vi "CSV_Image_Data_Append.vi"(0 "input cluster":T2={"Pinch-valve"="Test Sample", "XLP 6000 Pump"="MRJ", "Camera1"="", "Camera2"="", "Img_Capt"=FALSE, "Actuator"=FALSE, "Pump"=FALSE, "Cam 1"=FALSE, "Cam 2"=FALSE, "Empty_Refill"=FALSE, "Crop"=FALSE, "Light intensity"=0, "Exposure Time"=0.0, "Sample Name"="", "Operator"="", "Calibration 1"=path "C:/Users/au540322/Desktop/IHS_Project/images/Debris/Debris_0/Debris_0_2019_06_01-23-32-49-686.PNG", "Calibration 2"=path "C:/Users/au540322/Desktop/IHS_Project/images/Debris/Debris_0/Debris_0_2019_06_01-23-32-49-686.PNG", "Framerate"=1, "Timeout Sample"=1, "Collection date"="", "Sample size threshold"=10, "Empty start"=1, "Command"="", "Station"="", "Species Name"="", "Other Notes"="", "Aperture"=enum."Item 3", "Image Process Queue Size"=100, "Image Save Queue Size"=0, "Overload threshold"=0, "Max Framerate"=0, "Rectangle 1"={"Left"=0, "Top"=0, "Right"=0, "Bottom"=0, "Rotation"=0.0}, "Rectangle 2"={"Left"=0, "Top"=100, "Right"=100, "Bottom"=0, "Rotation"=0.0}, "Detection Region %"=200.0, "Detect 1"=path "C:/Users/au540322/Desktop/IHS_Project/images/Debris/Debris_0/Debris_0_2019_06_01-23-32-49-686.PNG", "Detect 2"=path "C:/Users/au540322/Desktop/IHS_Project/images/Debris/Debris_0/Debris_0_2019_06_01-23-32-49-686.PNG", "Max large object threshold"=500, "Open(T)/Close(F)"=FALSE, "Img_Capt Begin"=FALSE, "Dispense Speed"=0, "Flush Size"=0, "Location"="", "Latitude"="", "Longitude"="", "Determiner"="", "Sex"="", "Camera1_Img"=refnum, "Camera2_Img"=refnum, "Img1_Orig_Disp"=refnum, "Img2_Orig_Disp"=refnum, "Img1_Orig_RGB"=refnum, "Img2_Orig_RGB"=refnum, "Blue_Plane_Extract"=refnum, "Subtracted_Plane"=refnum, "Img1_Binary"=refnum, "Img2_Binary"=refnum, "Crop_Mask"=refnum, "Img1_Save"=refnum, "Img2_Save"=refnum, "Img1_Cali_Full"=refnum, "Img2_Cali_Full"=refnum, "Img1_Cali_Detect"=refnum, "Img2_Cali_Detect"=refnum, "Cam 1 queue"=refnum, "Cam 2 queue"=refnum, "Cam 1 - save queue"=refnum, "Cam 2 - save queue"=refnum, "Overlay_Ring"=0, "SystemVersion"=0, "System Serial"="", "Legacy Cam Attributes"=FALSE, "Camera Orientation 1"="", "Camera Orientation 2"="", "Pixel to mm 1"=0.0, "Pixel to mm 2"=0.0, "CAM1 Model"=enum."a2A5328-15ucBAS", "CAM2 Model"=enum."a2A5328-15ucBAS", "Flush Insect"=FALSE, "Pump Size"=FALSE} {"SystemVersion" items=["Standard", "XL"]; "Overlay_Ring" items=["Session Data", "Extended Setup", "Buffer", "Camera", "Dispenser", "Stats", "Connections"]; "Flush Size" min=1; "Dispense Speed" min=1; "Rectangle 2"."Rotation" format="%.2f"; "Rectangle 2"."Left" scale=0.0..1024.0; "Rectangle 2"."Right" scale=0.0..1024.0; "Rectangle 1"."Rotation" format="%.2f"; "Rectangle 1"."Left" scale=0.0..1024.0; "Rectangle 1"."Right" scale=0.0..1024.0; "Max Framerate" min=1; "Overload threshold" min=1; "Image Save Queue Size" min=1; "Image Process Queue Size" min=1; "Empty start" min=1; "Sample size threshold" min=1; "Framerate" min=1; "Light intensity" scale=0.0..100.0}, 1 "Image path":string, 2 "Sample Name":string, 3 "Image Name":string, 4 "Sample Data":dbl[](array[numeric]), 5 "ROI Descriptor":T1, 7 "Timestamp":string) -> ()   [LabVIEW 2024]
uses:
  controls/Data.ctl
  <vilib>/userDefined/High Color/IMAQdx.ctl
  <vilib>/vision/Image Controls.llb/IMAQ Image.ctl
  <vilib>/Utility/file.llb/Write Delimited Spreadsheet (string).vi
panel:
  out "string":string
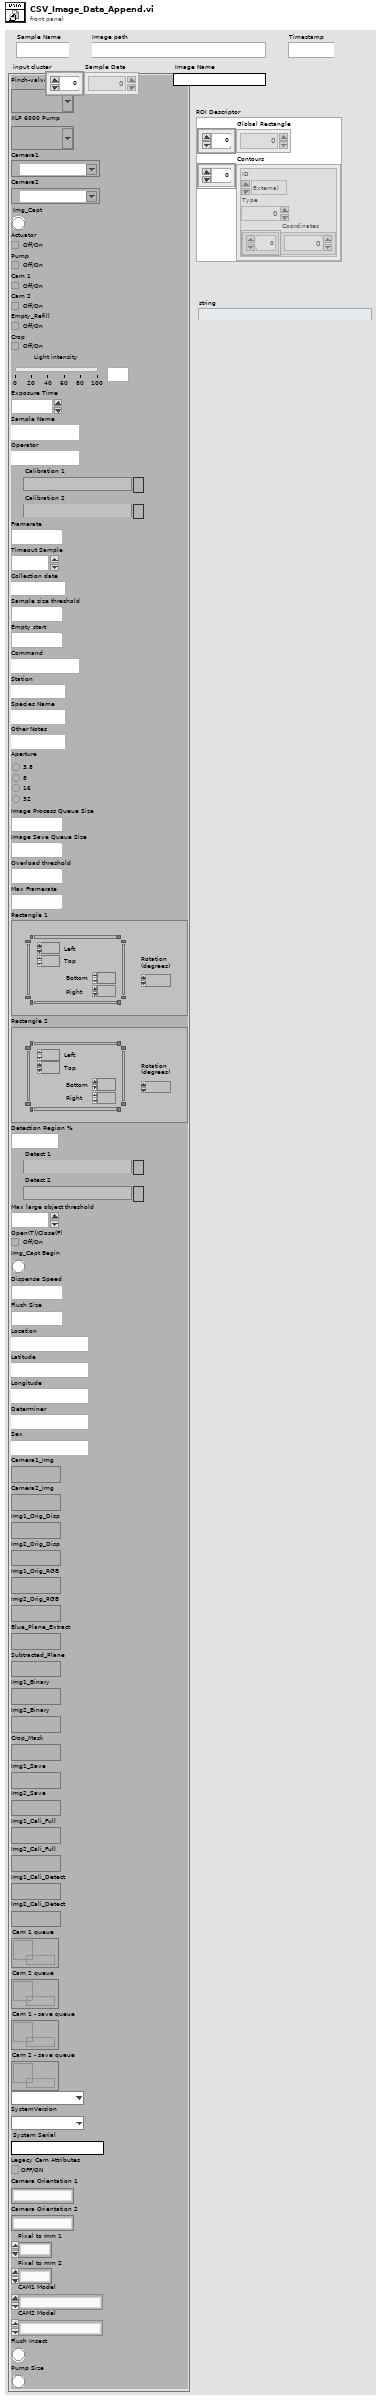
[diagram p1: front panel]
types:
  T1 = cluster{"Global Rectangle":i32[], "Contours":cluster{"ID":enum32{"External", "Internal"}, "Type":u32, "Coordinates":i32[]}[]}
  T2 = typedef "Data.ctl" = cluster{"Pinch-valve":refnum<visa-resource-name>, "XLP 6000 Pump":refnum<visa-resource-name>, "Camera1":T3, "Camera2":T3, "Img_Capt":bool, "Actuator":bool, "Pump":bool, "Cam 1":bool, "Cam 2":bool, "Empty_Refill":bool, "Crop":bool, "Light intensity":i32, "Exposure Time":dbl, "Sample Name":string, "Operator":string, "Calibration 1":path, "Calibration 2":path, "Framerate":i32, "Timeout Sample":i32, "Collection date":string, "Sample size threshold":i32, "Empty start":u32, "Command":string, "Station":string, "Species Name":string, "Other Notes":string, "Aperture":enum32{"Item 0", "Item 1", "Item 2", "Item 3"}, "Image Process Queue Size":i32, "Image Save Queue Size":i32, "Overload threshold":i32, "Max Framerate":i32, "Rectangle 1":T4, "Rectangle 2":T4, "Detection Region %":dbl, "Detect 1":path, "Detect 2":path, "Max large object threshold":i32, "Open(T)/Close(F)":bool, "Img_Capt Begin":bool, "Dispense Speed":i32, "Flush Size":i32, "Location":string, "Latitude":string, "Longitude":string, "Determiner":string, "Sex":string, "Camera1_Img":T5, "Camera2_Img":T5, "Img1_Orig_Disp":T5, "Img2_Orig_Disp":T5, "Img1_Orig_RGB":T5, "Img2_Orig_RGB":T5, "Blue_Plane_Extract":T5, "Subtracted_Plane":T5, "Img1_Binary":T5, "Img2_Binary":T5, "Crop_Mask":T5, "Img1_Save":T5, "Img2_Save":T5, "Img1_Cali_Full":T5, "Img2_Cali_Full":T5, "Img1_Cali_Detect":T5, "Img2_Cali_Detect":T5, "Cam 1 queue":refnum<queue>, "Cam 2 queue":refnum<queue>, "Cam 1 - save queue":refnum<queue>, "Cam 2 - save queue":refnum<queue>, "Overlay_Ring":u16, "SystemVersion":u16, "System Serial":string, "Legacy Cam Attributes":bool, "Camera Orientation 1":string, "Camera Orientation 2":string, "Pixel to mm 1":dbl, "Pixel to mm 2":dbl, "CAM1 Model":enum16{"a2A5328-15ucBAS", "acA1920-155uc"}, "CAM2 Model":enum16{"a2A5328-15ucBAS", "acA1920-155uc"}, "Flush Insect":bool, "Pump Size":bool}
  T3 = typedef "IMAQdx.ctl" = refnum<k21>
  T4 = typedef "IMAQ Rectangle" = cluster{"Left":i32, "Top":i32, "Right":i32, "Bottom":i32, "Rotation":dbl}
  T5 = typedef "IMAQ Image.ctl" = refnum<image>
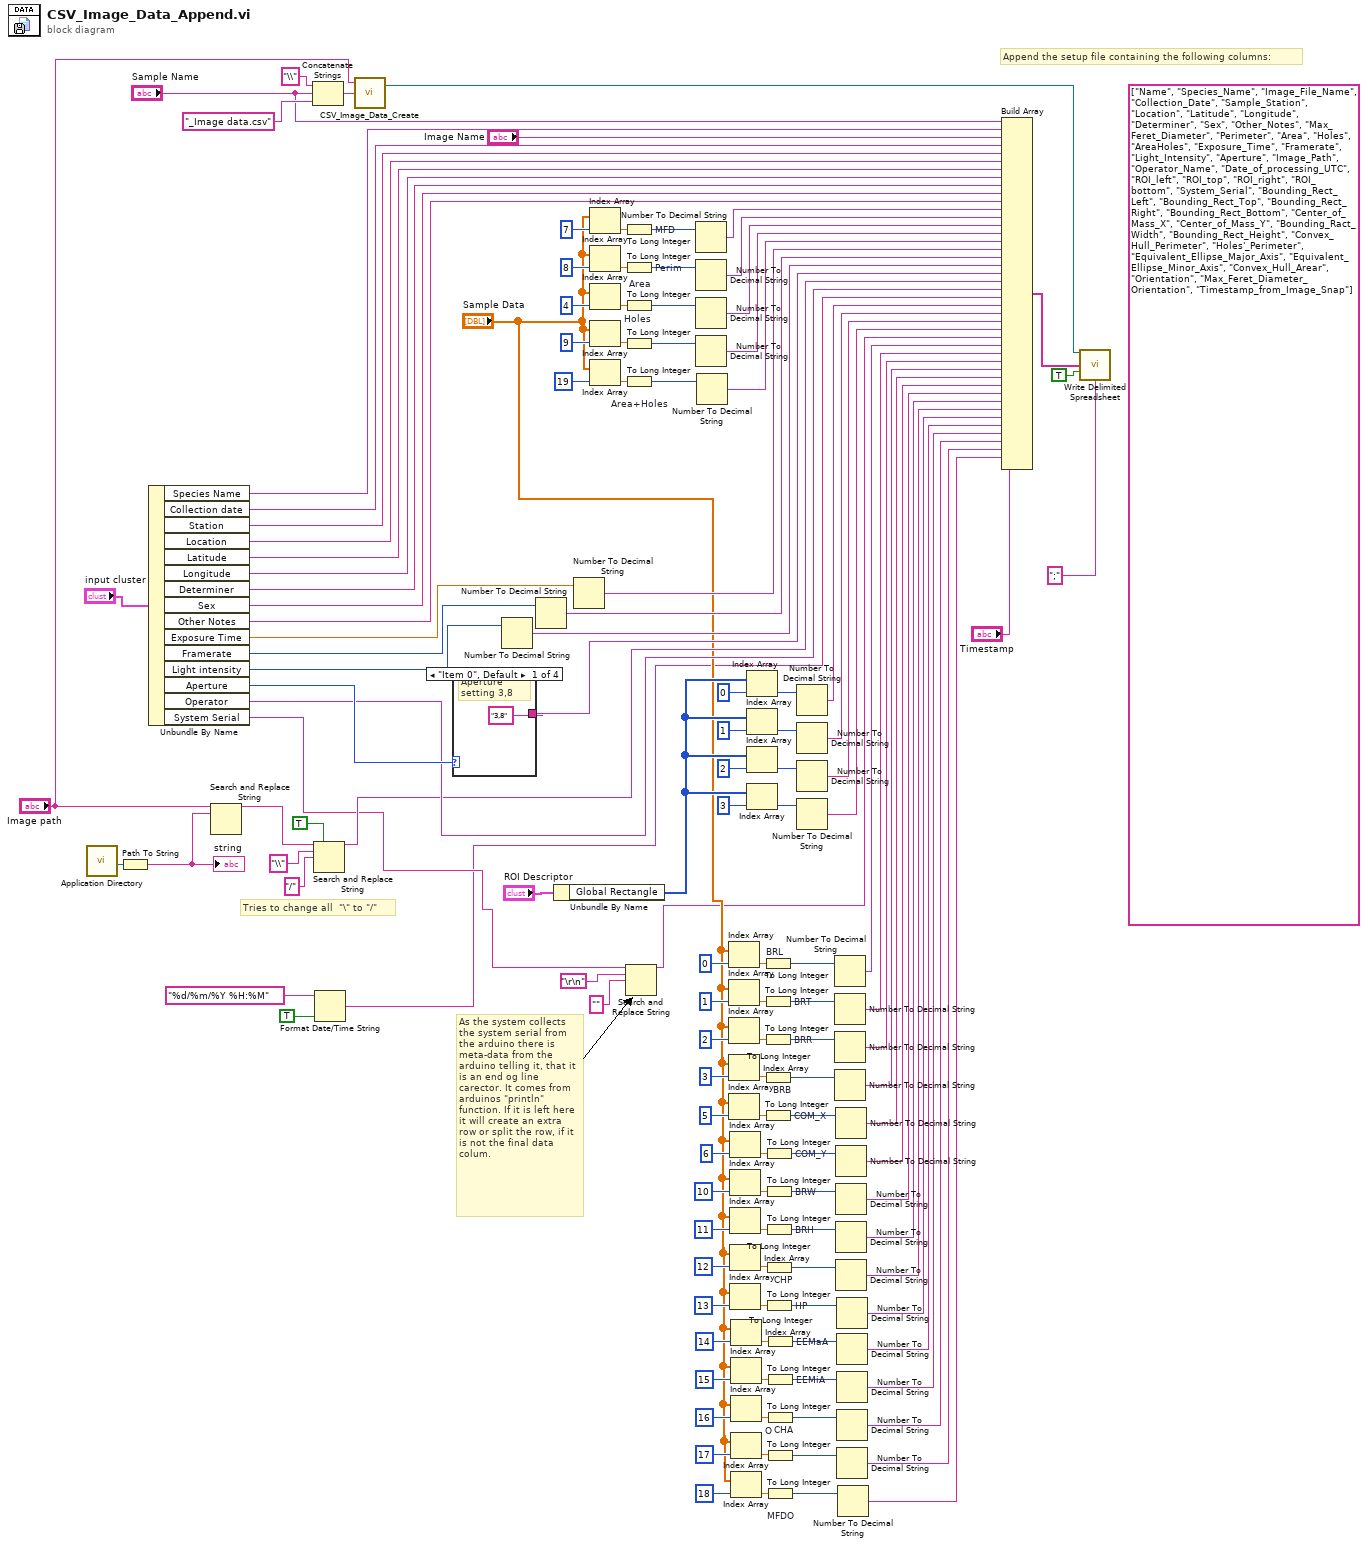
[diagram p0: block diagram]
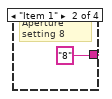
[diagram p2: hidden frame]
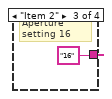
[diagram p3: hidden frame]
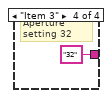
[diagram p4: hidden frame]
diagram:
  (unwired) string[] ["Name", "Species_Name", "Image_File_Name", "Collection_Date", "Sample_Station", "Location", "Latitude", "Longitude", "Determiner", "Sex", "Other_Notes", "Max_Feret_Diameter", "Perimeter", "Area", "Holes", "AreaHoles", "Exposure_Time", "Framerate", "Light_Intensity", "Aperture", "Image_Path", "Operator_Name", "Date_of_processing_UTC", "ROI_left", "ROI_top", "ROI_right", "ROI_bottom", "System_Serial", "Bounding_Rect_Left", "Bounding_Rect_Top", "Bounding_Rect_Right", "Bounding_Rect_Bottom", "Center_of_Mass_X", "Center_of_Mass_Y", "Bounding_Ract_Width", "Bounding_Rect_Height", "Convex_Hull_Perimeter", "Holes'_Perimeter", "Equivalent_Ellipse_Major_Axis", "Equivalent_Ellipse_Minor_Axis", "Convex_Hull_Arear", "Orientation", "Max_Feret_Diameter_Orientation", "Timestamp_from_Image_Snap"]
  # "As the system collects the system serial from the arduino there is meta-data from the arduino telling it, that it is an end og line carector. It comes from arduinos \"println\" function. If it is left here it will create an extra row or split the row, if it is not the final data colum."
  # "Tries to change all  \"\\\" to \"/\""
  # "Append the setup file containing the following columns:"
  n1 = call <vilib>:"Application Directory.vi"() -> ("Application Directory"=w136:path)
  n2 = Path To String(path=w136) -> (string=w135:string)
  "string" <- w135
  n3 = Unbundle By Name("input cluster") -> ("Species Name"=w118:string, "Collection date"=w119:string, "Station"=w120:string, "Location"=w121:string, "Latitude"=w122:string, "Longitude"=w123:string, "Determiner"=w124:string, "Sex"=w125:string, "Other Notes"=w126:string, "Exposure Time"=w134:dbl, "Framerate"=w80:i32, "Light intensity"=w133:i32, "Aperture"=w132:enum32{"Item 0", "Item 1", "Item 2", "Item 3"}, "Operator"=w127:string, "System Serial"=w21:string)
  n4 = Search and Replace String(input string="Image path", search string=w135) -> (result string=w68:string)  [unwired: 6 in, 3 out]
  n5 = Concatenate Strings("\\" ("string"), "Sample Name", "_Image data.csv") -> (w75:string)
  n6 = Search and Replace String(replace all?=TRUE ("replace all? (F)"), input string=w68, search string="\\", replace string="/" ("replace string (\"\")")) -> (result string=w69:string)  [unwired: 4 in, 3 out]
  n7 = Format Date/Time String(time format string (%c)="%d/%m/%Y %H:%M", UTC format=TRUE) -> (date/time string=w2:string)  [unwired: 1 in]
  n8 = call "CSV_Image_Data_Create.vi"("File name"=w75, "Image path"="Image path") -> ("Image data file"=w74:path)  [unwired: 2 in, 1 out]
  n9 = case shown="\"Item 0\", Default" w132 {
    tunnel: ["3,8" "8" "16" "32"] -> w128
    frame "Item 0", Default {
      # "Aperture setting 3,8"
    }
    frame "Item 1" {
      # "Aperture setting 8"
    }
    frame "Item 2" {
      # "Aperture setting 16"
    }
    frame "Item 3" {
      # "Aperture setting 32"
    }
  }
  n10 = Number To Decimal String(number=w133) -> (decimal integer string=w129:string)  [unwired: 1 in]
  n11 = Number To Decimal String(number=w80) -> (decimal integer string=w130:string)  [unwired: 1 in]
  n12 = Unbundle By Name("ROI Descriptor") -> ("Global Rectangle"=w85:i32[])
  n13 = Number To Decimal String(number=w134) -> (decimal integer string=w131:string)  [unwired: 1 in]
  n14 = Index Array ("MFD")(array="Sample Data", index=7) -> (element=w109:dbl)
  n15 = Index Array ("MFD")(array="Sample Data", index=8) -> (element=w104:dbl)
  n16 = Index Array ("MFD")(array="Sample Data", index=4) -> (element=w102:dbl)
  n17 = Index Array ("MFD")(array="Sample Data", index=9) -> (element=w103:dbl)
  n18 = Index Array ("MFD")(array="Sample Data", index=19) -> (element=w101:dbl)
  n19 = To Long Integer "MFD"(number=w109) -> (32bit integer=w115:i32)
  n20 = To Long Integer "Perim"(number=w104) -> (32bit integer=w114:i32)
  n21 = To Long Integer "Area"(number=w102) -> (32bit integer=w113:i32)
  n22 = To Long Integer "Holes"(number=w103) -> (32bit integer=w112:i32)
  n23 = To Long Integer "Area+Holes"(number=w101) -> (32bit integer=w111:i32)
  n24 = Search and Replace String(input string=w21, search string="\r\n", replace string="" ("replace string (\"\")")) -> (result string=w18:string)  [unwired: 5 in, 3 out]
  n25 = Number To Decimal String(number=w115) -> (decimal integer string=w100:string)  [unwired: 1 in]
  n26 = Number To Decimal String(number=w114) -> (decimal integer string=w99:string)  [unwired: 1 in]
  n27 = Number To Decimal String(number=w113) -> (decimal integer string=w98:string)  [unwired: 1 in]
  n28 = Number To Decimal String(number=w112) -> (decimal integer string=w97:string)  [unwired: 1 in]
  n29 = Number To Decimal String(number=w111) -> (decimal integer string=w96:string)  [unwired: 1 in]
  n30 = Index Array ("MFD")(array="Sample Data", index=0) -> (element=w61:dbl)
  n31 = Index Array ("MFD")(array="Sample Data", index=1) -> (element=w56:dbl)
  n32 = Index Array ("MFD")(array="Sample Data", index=2) -> (element=w54:dbl)
  n33 = Index Array ("MFD")(array="Sample Data", index=3) -> (element=w55:dbl)
  n34 = Index Array ("MFD")(array="Sample Data", index=5) -> (element=w53:dbl)
  n35 = Index Array ("MFD")(array="Sample Data", index=6) -> (element=w46:dbl)
  n36 = Index Array ("MFD")(array="Sample Data", index=10) -> (element=w41:dbl)
  n37 = Index Array ("MFD")(array="Sample Data", index=11) -> (element=w39:dbl)
  n38 = Index Array ("MFD")(array="Sample Data", index=12) -> (element=w40:dbl)
  n39 = Index Array ("MFD")(array="Sample Data", index=13) -> (element=w38:dbl)
  n40 = Index Array ("MFD")(array="Sample Data", index=14) -> (element=w31:dbl)
  n41 = Index Array ("MFD")(array="Sample Data", index=15) -> (element=w26:dbl)
  n42 = Index Array ("MFD")(array="Sample Data", index=16) -> (element=w24:dbl)
  n43 = Index Array ("MFD")(array="Sample Data", index=17) -> (element=w25:dbl)
  n44 = Index Array ("MFD")(array="Sample Data", index=18) -> (element=w23:dbl)
  n45 = Index Array ("MFD")(array=w85, index=0) -> (element=w93:i32)
  n46 = Index Array ("MFD")(array=w85, index=1) -> (element=w92:i32)
  n47 = Index Array ("MFD")(array=w85, index=2) -> (element=w91:i32)
  n48 = Index Array ("MFD")(array=w85, index=3) -> (element=w90:i32)
  n49 = To Long Integer "BRL"(number=w61) -> (32bit integer=w67:i32)
  n50 = To Long Integer "BRT"(number=w56) -> (32bit integer=w66:i32)
  n51 = To Long Integer "BRR"(number=w54) -> (32bit integer=w65:i32)
  n52 = To Long Integer "BRB"(number=w55) -> (32bit integer=w64:i32)
  n53 = To Long Integer "COM_X"(number=w53) -> (32bit integer=w63:i32)
  n54 = To Long Integer "COM_Y"(number=w46) -> (32bit integer=w52:i32)
  n55 = To Long Integer "BRW"(number=w41) -> (32bit integer=w51:i32)
  n56 = To Long Integer "BRH"(number=w39) -> (32bit integer=w50:i32)
  n57 = To Long Integer "CHP"(number=w40) -> (32bit integer=w49:i32)
  n58 = To Long Integer "HP"(number=w38) -> (32bit integer=w48:i32)
  n59 = To Long Integer "EEMaA"(number=w31) -> (32bit integer=w37:i32)
  n60 = To Long Integer "EEMiA"(number=w26) -> (32bit integer=w36:i32)
  n61 = To Long Integer "CHA"(number=w24) -> (32bit integer=w35:i32)
  n62 = To Long Integer "O"(number=w25) -> (32bit integer=w34:i32)
  n63 = To Long Integer "MFDO"(number=w23) -> (32bit integer=w33:i32)
  n64 = Number To Decimal String(number=w93) -> (decimal integer string=w84:string)  [unwired: 1 in]
  n65 = Number To Decimal String(number=w92) -> (decimal integer string=w83:string)  [unwired: 1 in]
  n66 = Number To Decimal String(number=w91) -> (decimal integer string=w82:string)  [unwired: 1 in]
  n67 = Number To Decimal String(number=w90) -> (decimal integer string=w81:string)  [unwired: 1 in]
  n68 = Number To Decimal String(number=w67) -> (decimal integer string=w17:string)  [unwired: 1 in]
  n69 = Number To Decimal String(number=w66) -> (decimal integer string=w16:string)  [unwired: 1 in]
  n70 = Number To Decimal String(number=w65) -> (decimal integer string=w15:string)  [unwired: 1 in]
  n71 = Number To Decimal String(number=w64) -> (decimal integer string=w14:string)  [unwired: 1 in]
  n72 = Number To Decimal String(number=w63) -> (decimal integer string=w13:string)  [unwired: 1 in]
  n73 = Number To Decimal String(number=w52) -> (decimal integer string=w12:string)  [unwired: 1 in]
  n74 = Number To Decimal String(number=w51) -> (decimal integer string=w11:string)  [unwired: 1 in]
  n75 = Number To Decimal String(number=w50) -> (decimal integer string=w10:string)  [unwired: 1 in]
  n76 = Number To Decimal String(number=w49) -> (decimal integer string=w9:string)  [unwired: 1 in]
  n77 = Number To Decimal String(number=w48) -> (decimal integer string=w8:string)  [unwired: 1 in]
  n78 = Number To Decimal String(number=w37) -> (decimal integer string=w7:string)  [unwired: 1 in]
  n79 = Number To Decimal String(number=w36) -> (decimal integer string=w6:string)  [unwired: 1 in]
  n80 = Number To Decimal String(number=w35) -> (decimal integer string=w5:string)  [unwired: 1 in]
  n81 = Number To Decimal String(number=w34) -> (decimal integer string=w4:string)  [unwired: 1 in]
  n82 = Number To Decimal String(number=w33) -> (decimal integer string=w3:string)  [unwired: 1 in]
  n83 = Build Array("Sample Name", w118, "Image Name", w119, w120, w121, w122, w123, w124, w125, w126, w100, w99, w98, w97, w96, w131, w130, w129, w128, w69, w127, w2, w84, w83, w82, w81, w18, w17, w16, w15, w14, w13, w12, w11, w10, w9, w8, w7, w6, w5, w4, w3, "Timestamp") -> (w116:string[])
  n84 = call-poly <vilib>:"Write Delimited Spreadsheet.vi"("file path (dialog if empty)"=w74, "1D data"=w116, "append to file? (new file:F)"=TRUE, "delimiter (\\t)"=";" ("delimiter (\\t)")) -> ()  [unwired: 10 in, 2 out]
